vi "Caller.vi"(0 "Add in":refnum<class "Add.lvclass">, 2 "DVR":refnum<data-value>, 5 "Sub Panel":refnum<vi>, 7 "User Event Ref":refnum<user-event>, 11 "Error In":errorcluster) -> (4 "Add out":refnum<class "Add.lvclass">, 15 "Error Out":errorcluster)   [LabVIEW 2023, in "Add.lvclass"]
doc: "The VI asynchronously calls the Operation UI method of the addition operation."
uses:
  Add.lvclass
  C:/Users/Ancy.Augustin/Downloads/LVOOPS DVR/LVOOPS DVR/Classes/Arithemtic Operation/Arithemetic Operation.lvclass
  Arithemtic Operation/Arithemetic Operation.lvclass
  Typedef/User Event Data.ctl
  Operation UI.vi
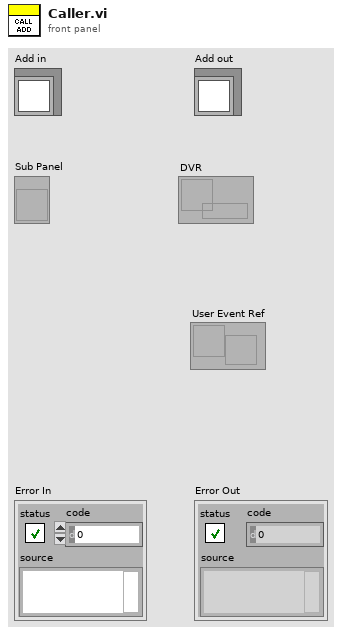
[diagram p1: front panel]
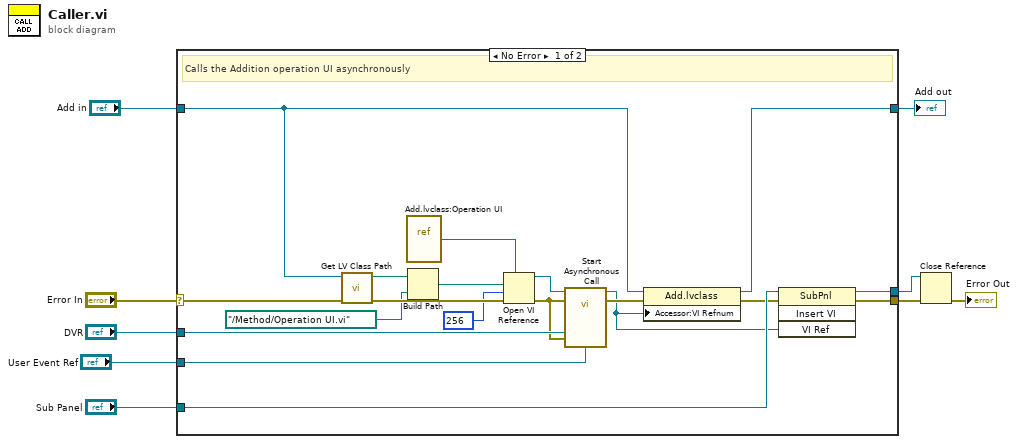
[diagram p0: block diagram]
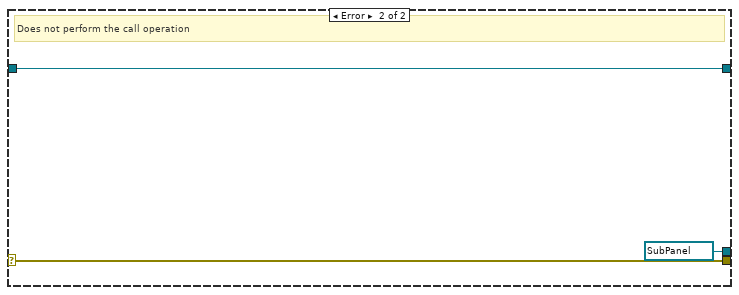
[diagram p2: hidden frame]
diagram:
  n1 = case shown="No Error" "Error In" {
    selector: "Error In" -> [w22 w31]
    tunnel: [w21 w31] -> w8
    tunnel: [w16 w30] -> w6
    tunnel: "Add in" -> [w15 w30]
    tunnel: "Sub Panel" -> [w20 _]
    tunnel: [w19 refnum<vi> refnum ("Sub Panel")] -> w3
    tunnel: "DVR" -> [w12 _]
    tunnel: "User Event Ref" -> [w10 _]
    frame No Error {
      # "Calls the Addition operation UI asynchronously"
      n2 = call <vilib>:"Get LV Class Path.vi"("error in (no error)"=w22, "object"=w15) -> ("error out"=w28:errorcluster, "class path"=w27:path)  [unwired: 8 in]
      n3 = vi-ref "Add.lvclass:Operation UI.vi"() -> (w14:refnum<vi>)
      n4 = Build Path(base path=w27, name or relative path=path "../Method/Operation UI.vi") -> (appended path=w13:path)
      n5 = Open VI Reference(type specifier VI Refnum (for type only)=w14, vi path=w13, options=256, error in (no error)=w28) -> (vi reference=w23:refnum<vi>, error out=w11:errorcluster)  [unwired: 2 in]
      n6 = call-by-ref "Start Asynchronous Call"(reference=w23, error in=w11, "DVR In"=w12, "Error In"=w11, "User Event Ref"=w10) -> (reference out=w17:refnum<vi>, error out=w25:errorcluster)  [unwired: 10 in, 3 out]
      n7 = property class="Add.lvclass"(reference=w15, error in=w25, "Accessor:VI Refnum"=w17) -> (reference out=w16:refnum<class "Add.lvclass">, error out=w18:errorcluster)
      n8 = invoke class="SubPnl" method="Insert VI"(reference=w20, error in=w18, "VI Ref"=w17) -> (reference out=w19:refnum<vi>, error out=w21:errorcluster)  [unwired: 1 in, 2 out]
    }
    frame Error {
      # "Does not perform the call operation"
    }
  }
  "Add out" <- w6
  n9 = Close Reference(reference=w3, error in (no error)=w8) -> (error out=→"Error Out":errorcluster)
